vi "Build Check Low Priority Time.vi"(6 "Group":i32, 7 "Virtual Memory Unit in":refnum<class "Virtual Memory Unit.lvclass">, 8 "error in (no error)":errorcluster, 10 "Starting Address":u16 format="%04x", 11 "Major Frame in":refnum<class "Major Frame.lvclass">) -> (0 "error out":errorcluster, 2 "Next Available Address":u16 format="%04x", 3 "Major Frame out":refnum<class "Major Frame.lvclass">, 5 "Virtual Memory Unit out":refnum<class "Virtual Memory Unit.lvclass">)   [LabVIEW 2016, in "BCI-1553 API.lvlib" / "Major Frame.lvclass"]
doc: "Checks if there's enough time to run a low-priority async message."
uses:
  Major Frame.lvclass
  TypeDefs/BC Condition Codes.ctl
  BCI-1553 API.lvlib
  TypeDefs/BC Op Codes - Verbose.ctl
  Dependencies/Virtual Memory Unit/Virtual Memory Unit.lvclass
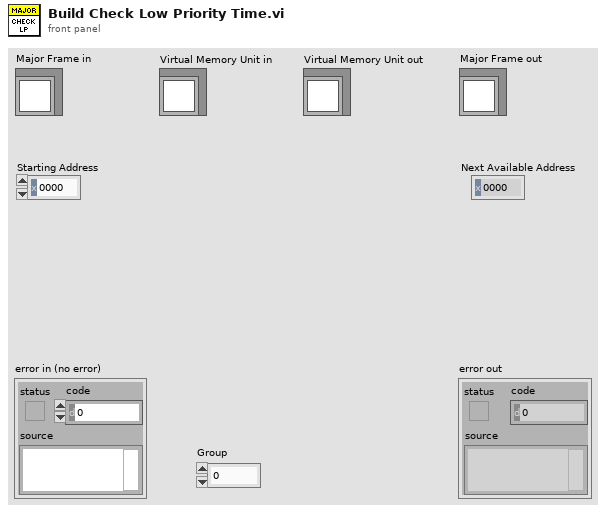
[diagram p1: front panel]
types:
  T1 = typedef "BCI-1553 API.lvlib/BC Op Codes - Verbose.ctl" = enum16{"EXECUTE MSG", "EXECUTE MSG GO", "JUMP", "CALL SUBROUTINE", "RETURN", "INTERRUPT REQUEST", "HALT", "DELAY", "WAIT FRAME TIMER = 0", "COMPARE FRAME TIMER", "COMPARE MSG TIMER", "LOAD TIME TAG CTR", "LOAD TIME TAG CTR HI", "LOAD FRAME TIMER", "START FRAME TIMER", "PUSH TIME TAG COUNT", "PUSH TIME TAG COUNT HI", "PUSH TIME TAG COUNT BOTH", "PUSH BLOCK STATUS WORD", "PUSH CURRENT VALUE", "PUSH INDIRECT", "WAIT EXT TRIGGER", "EXECUTE AND FLIP", "EXECUTE, FLIP, GO", "WRITE VALUE TO WMI", "WRITE VALUE TO MEM", "DECREMENT RAM, SKIP", "FLAG"}
  T2 = typedef "BCI-1553 API.lvlib/BC Condition Codes.ctl" = enum16{"GP0 == 1 || LT", "GP1 == 1 || NE", "GP2 == 1", "GP3 == 1", "GP4 == 1", "GP5 == 1", "GP6 == 1", "GP7 == 1", "NORESP", "FMTERR", "GOODBLOCK", "MSKSTATSET", "BADMSG", "1RETRY", "2RETRY", "ALWAYS"}
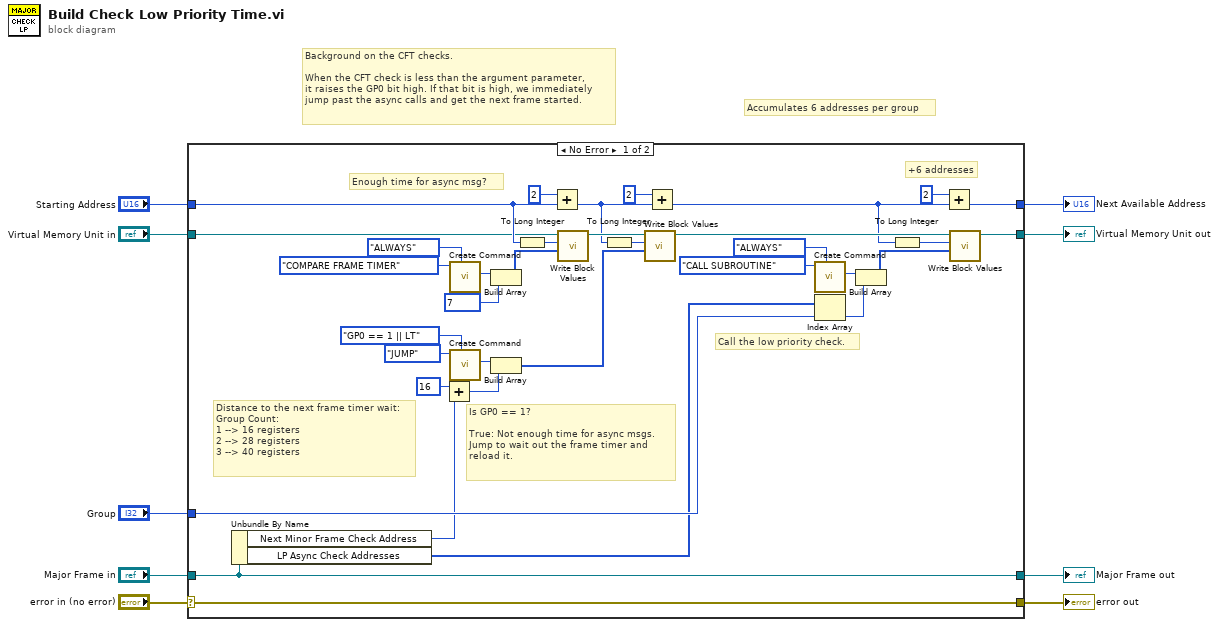
[diagram p0: block diagram]
diagram:
  # "Background on the CFT checks.\n\nWhen the CFT check is less than the argument parameter,\nit raises the GP0 bit high. If that bit is high, we immediately\njump past the async calls and get the next frame started."
  # "Accumulates 6 addresses per group"
  n1 = case shown="No Error" "error in (no error)" {
    selector: "error in (no error)" -> [w44 w48]
    tunnel: [w44 w48] -> w8
    tunnel: [w11 w47] -> w6
    tunnel: "Major Frame in" -> [w11 w47]
    tunnel: "Virtual Memory Unit in" -> [w14 w45]
    tunnel: [w16 w46] -> w4
    tunnel: "Starting Address" -> [w17 w46]
    tunnel: "Group" -> [w15 _]
    tunnel: [w13 w45] -> w1
    frame No Error {
      # "Distance to the next frame timer wait:\nGroup Count:\n1 --> 16 registers\n2 --> 28 registers\n3 --> 40 registers"
      # "Enough time for async msg?"
      # "+6 addresses"
      # "Call the low priority check."
      # "Is GP0 == 1?\n\nTrue: Not enough time for async msgs.\nJump to wait out the frame timer and\nreload it."
      n2 = Unbundle By Name(w11) -> ("Next Minor Frame Check Address"=w12:u16, "LP Async Check Addresses"=w10:u16[])
      n3 = Add(x=u16 16 ("element"), y=w12) -> (x+y=w19:u16)
      n4 = call "Create Command.vi"("Condition"=BC_Condition_Codes."ALWAYS", "Op Code"=BC_Op_Codes_-_Verbose."COMPARE FRAME TIMER") -> ("Instruction"=w32:u16)  [unwired: 8 in, 1 out]
      n5 = call "Create Command.vi"("Condition"=BC_Condition_Codes."GP0 == 1 || LT", "Op Code"=BC_Op_Codes_-_Verbose."JUMP") -> ("Instruction"=w26:u16)  [unwired: 8 in, 1 out]
      n6 = Build Array(w32, u16 7 ("element")) -> (w30:u16[])
      n7 = Build Array(w26, w19) -> (w27:u16[])
      n8 = To Long Integer(number=w17) -> (32bit integer=w29:i32)
      n9 = Add(x=u16 2, y=w17) -> (x+y=w22:u16)
      n10 = call "Write Block Values.vi"("Write Block"=w30, "Start Index"=w29, "Virtual Memory Unit in"=w14) -> ("Virtual Memory Unit out"=w23:refnum<class "Virtual Memory Unit.lvclass">)  [unwired: 7 in, 1 out]
      n11 = To Long Integer(number=w22) -> (32bit integer=w28:i32)
      n12 = call "Write Block Values.vi"("Write Block"=w27, "Start Index"=w28, "Virtual Memory Unit in"=w23) -> ("Virtual Memory Unit out"=w43:refnum<class "Virtual Memory Unit.lvclass">)  [unwired: 7 in, 1 out]
      n13 = Add(x=u16 2, y=w22) -> (x+y=w42:u16)
      n14 = call "Create Command.vi"("Condition"=BC_Condition_Codes."ALWAYS", "Op Code"=BC_Op_Codes_-_Verbose."CALL SUBROUTINE") -> ("Instruction"=w38:u16)  [unwired: 8 in, 1 out]
      n15 = Index Array(array=w10, index=w15) -> (element=w36:u16)
      n16 = Build Array(w38, w36) -> (w37:u16[])
      n17 = To Long Integer(number=w42) -> (32bit integer=w41:i32)
      n18 = Add(x=u16 2, y=w42) -> (x+y=w16:u16)
      n19 = call "Write Block Values.vi"("Write Block"=w37, "Start Index"=w41, "Virtual Memory Unit in"=w43) -> ("Virtual Memory Unit out"=w13:refnum<class "Virtual Memory Unit.lvclass">)  [unwired: 7 in, 1 out]
    }
    frame Error {
    }
  }
  "error out" <- w8
  "Major Frame out" <- w6
  "Virtual Memory Unit out" <- w1
  "Next Available Address" <- w4
